vi "Drive Test.vi"(11 "Pilot-CoPilot Gamepad Controls":T1) -> ()   [LabVIEW 2014]
uses:
  Subsystems VIs/Robot Control Outputs 2015.ctl
  Global Variables/Refnum Names.vi
panel:
  # "CB = control board"
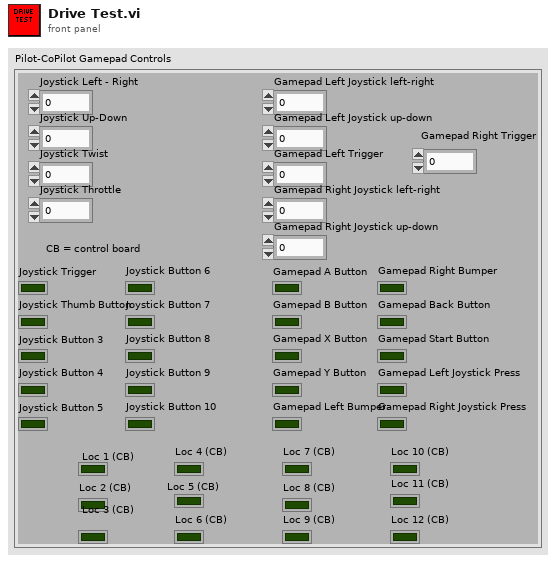
[diagram p1: front panel]
types:
  T1 = typedef "Robot Control Outputs 2015.ctl" = cluster{"Gamepad Left Joystick left-right":dbl, "Gamepad Left Joystick up-down":dbl, "Gamepad A Button":bool, "Gamepad B Button":bool, "Gamepad X Button":bool, "Gamepad Y Button":bool, "Gamepad Left Bumper":bool, "Gamepad Right Bumper":bool, "Gamepad Back Button":bool, "Gamepad Start Button":bool, "Gamepad Left Joystick Press":bool, "Gamepad Right Joystick Press":bool, "Joystick Trigger":bool, "Joystick Thumb Button":bool, "Joystick Button 3":bool, "Joystick Button 4":bool, "Joystick Button 5":bool, "Joystick Button 6":bool, "Joystick Button 7":bool, "Joystick Button 8":bool, "Joystick Button 9":bool, "Joystick Button 10":bool, "Gamepad Left Trigger":dbl, "Gamepad Right Joystick left-right":dbl, "Gamepad Right Joystick up-down":dbl, "Joystick Left - Right":dbl, "Joystick Up-Down":dbl, "Joystick Twist":dbl, "Joystick Throttle":dbl, "Loc 1 (CB)":bool, "Loc 4 (CB)":bool, "Gamepad Right Trigger":dbl, "Loc 2 (CB)":bool, "Loc 3 (CB)":bool, "Loc 5 (CB)":bool, "Loc 6 (CB)":bool, "Loc 7 (CB)":bool, "Loc 10 (CB)":bool, "Loc 8 (CB)":bool, "Loc 9 (CB)":bool, "Loc 11 (CB)":bool, "Loc 12 (CB)":bool}
  T2 = typedef "WPI_MotorControlDeviceRef.ctl" = cluster{"DeviceStatus":errorcluster, "Type":T3, "PWM":cluster{"Controller":T4, "PWM Channel":T5, "DeadBand":T6}, "CAN":cluster{"Device Number":u8, "Control Mode":T7, "Semaphore":T8, "Max Vout":dbl, "TalonSRX Control Mode":T9}, "Invert":bool, "TransformRef":T10, "InvTransformRef":T10}
  T3 = typedef "WPI_MotorControlType.ctl" = enum16{"PWM", "CAN", "CANTalonSRX"}
  T4 = typedef "FPGA_TypedefDigitalModule.ctl" = enum16{"Controller 1"}
  T5 = typedef "FPGA_DIOPWMChannel.ctl" = enum8{"PWM 0", "PWM 1", "PWM 2", "PWM 3", "PWM 4", "PWM 5", "PWM 6", "PWM 7", "PWM 8", "PWM 9", "PWM MXP 0", "PWM MXP 1", "PWM MXP 2", "PWM MXP 3", "PWM MXP 4", "PWM MXP 5", "PWM MXP 6", "PWM MXP 7", "PWM MXP 8", "PWM MXP 9", "Invalid"}
  T6 = typedef "WPI_PWMDeadband.ctl" = cluster{"Name":string, "maxPositivePwm":i32, "minPositivePwm":i32, "centerPwm":i32, "maxNegativePwm":i32, "minNegativePwm":i32, "angularRange":u16}
  T7 = typedef "WPI_CANJaguar_ControlMode.ctl" = enum8{"Percent VBus", "Current", "Speed", "Position", "Voltage"}
  T8 = typedef "Semaphore RefNum" = refnum<k1>
  T9 = typedef "WPI_CANTalonSRX_APIControlMode.ctl" = enum8{"Percent VBus", "Speed", "Position", "Slave", "Unchanged / Invalid"}
  T10 = typedef "WPI_PWMTransform_ConPane.ctl" = refnum<vi>
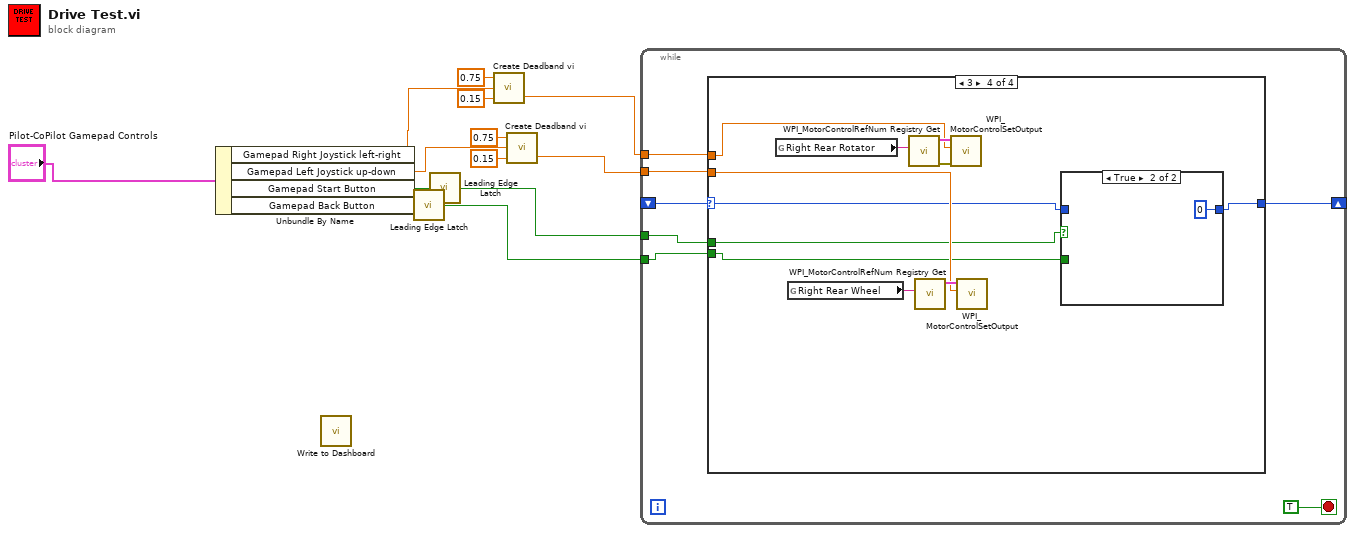
[diagram p0: block diagram]
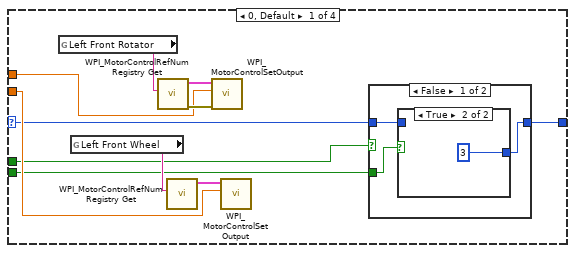
[diagram p2: hidden frame]
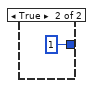
[diagram p4: hidden frame]
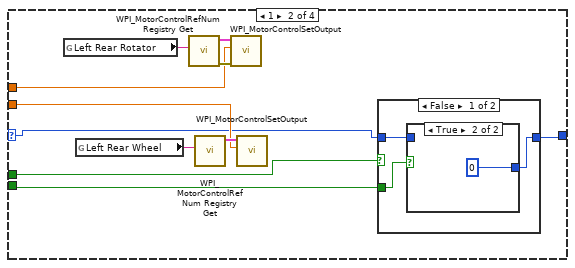
[diagram p5: hidden frame]
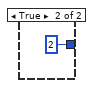
[diagram p7: hidden frame]
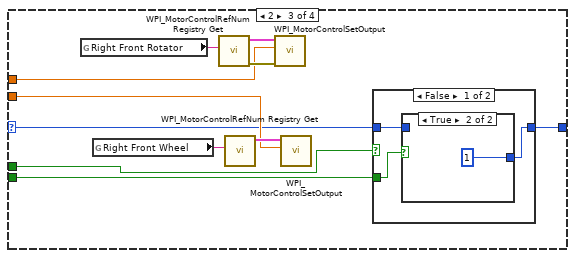
[diagram p8: hidden frame]
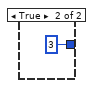
[diagram p10: hidden frame]
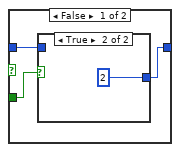
[diagram p11: hidden frame]
diagram:
  n1 = Unbundle By Name("Pilot-CoPilot Gamepad Controls") -> ("Gamepad Right Joystick left-right"=w8:dbl, "Gamepad Left Joystick up-down"=w2:dbl, "Gamepad Start Button"=w12:bool, "Gamepad Back Button"=w11:bool)
  n2 = call "Write to Dashboard.vi"() -> ()  [unwired: 12 in]
  n3 = call "Leading Edge Latch.vi"("Input"=w11) -> ("Output"=w10:bool)
  n4 = call "Leading Edge Latch.vi"("Input"=w12) -> ("Output"=w9:bool)
  n5 = call "Create Deadband vi.vi"("Input Deadband"=0.15, "Input"=w8, "Output Upper Limit"=0.75) -> ("Output"=w5:dbl)  [unwired: 1 in]
  n6 = call "Create Deadband vi.vi"("Input Deadband"=0.15, "Input"=w2, "Output Upper Limit"=0.75) -> ("Output"=w1:dbl)  [unwired: 1 in]
  n7 = while {
    tunnel: w5 -> [w20]
    tunnel: w1 -> [w19]
    shift-right: [w17] -> _
    shift-left: _ -> [w16]
    tunnel: w9 -> [w15]
    tunnel: w10 -> [w14]
    stop <- TRUE stop-if-true
    n8 = case shown="3" w16 {
      selector: w16 -> [w23 w38 w57 w74]
      tunnel: w20 -> [w26 w43 w60 w77]
      tunnel: w19 -> [w25 w42 w59 w76]
      tunnel: [w22 w41 w58 w75] -> w17
      tunnel: w15 -> [w24 w39 w56 w73]
      tunnel: w14 -> [w21 w40 w55 w72]
      frame 0, Default {
        n9 = global read "Refnum Names.vi" "Left Front Rotator"() -> (w31:string)
        n10 = global read "Refnum Names.vi" "Left Front Wheel"() -> (w28:string)
        n11 = call <vilib>:"WPI_MotorControlRefNum Registry Get.vi"("refnum name"=w31) -> ("error out"=w29:errorcluster, "MotorControlDevRef"=w30:T2)  [unwired: 9 in]
        n12 = call <vilib>:"WPI_MotorControlRefNum Registry Get.vi"("refnum name"=w28) -> ("MotorControlDevRef"=w27:T2)  [unwired: 9 in, 1 out]
        n13 = call <vilib>:"WPI_MotorControlSetOutput.vi"("error in (no error)"=w29, "Output"=w26, "MotorControlDevRef"=w30) -> ()  [unwired: 6 in, 3 out]
        n14 = call <vilib>:"WPI_MotorControlSetOutput.vi"("Output"=w25, "MotorControlDevRef"=w27) -> ()  [unwired: 7 in, 3 out]
        n15 = case shown="False" w24 {
          tunnel: w23 -> [w32 _]
          tunnel: [w33 1] -> w22
          tunnel: w21 -> [w34 _]
          frame False {
            n16 = case shown="True" w34 {
              tunnel: [w35 3] -> w33
              tunnel: w32 -> [w35 _]
              frame False {
              }
              frame True {
              }
            }
          }
          frame True {
          }
        }
      }
      frame 1 {
        n17 = global read "Refnum Names.vi" "Left Rear Rotator"() -> (w48:string)
        n18 = global read "Refnum Names.vi" "Left Rear Wheel"() -> (w45:string)
        n19 = call <vilib>:"WPI_MotorControlRefNum Registry Get.vi"("refnum name"=w48) -> ("error out"=w46:errorcluster, "MotorControlDevRef"=w47:T2)  [unwired: 9 in]
        n20 = call <vilib>:"WPI_MotorControlRefNum Registry Get.vi"("refnum name"=w45) -> ("MotorControlDevRef"=w44:T2)  [unwired: 9 in, 1 out]
        n21 = call <vilib>:"WPI_MotorControlSetOutput.vi"("error in (no error)"=w46, "Output"=w43, "MotorControlDevRef"=w47) -> ()  [unwired: 6 in, 3 out]
        n22 = call <vilib>:"WPI_MotorControlSetOutput.vi"("Output"=w42, "MotorControlDevRef"=w44) -> ()  [unwired: 7 in, 3 out]
        n23 = case shown="False" w39 {
          tunnel: w38 -> [w49 _]
          tunnel: [w50 2] -> w41
          tunnel: w40 -> [w51 _]
          frame False {
            n24 = case shown="True" w51 {
              tunnel: [w52 0] -> w50
              tunnel: w49 -> [w52 _]
              frame False {
              }
              frame True {
              }
            }
          }
          frame True {
          }
        }
      }
      frame 2 {
        n25 = global read "Refnum Names.vi" "Right Front Rotator"() -> (w65:string)
        n26 = global read "Refnum Names.vi" "Right Front Wheel"() -> (w62:string)
        n27 = call <vilib>:"WPI_MotorControlRefNum Registry Get.vi"("refnum name"=w65) -> ("error out"=w63:errorcluster, "MotorControlDevRef"=w64:T2)  [unwired: 9 in]
        n28 = call <vilib>:"WPI_MotorControlRefNum Registry Get.vi"("refnum name"=w62) -> ("MotorControlDevRef"=w61:T2)  [unwired: 9 in, 1 out]
        n29 = call <vilib>:"WPI_MotorControlSetOutput.vi"("error in (no error)"=w63, "Output"=w60, "MotorControlDevRef"=w64) -> ()  [unwired: 6 in, 3 out]
        n30 = call <vilib>:"WPI_MotorControlSetOutput.vi"("Output"=w59, "MotorControlDevRef"=w61) -> ()  [unwired: 7 in, 3 out]
        n31 = case shown="False" w56 {
          tunnel: w57 -> [w66 _]
          tunnel: [w67 3] -> w58
          tunnel: w55 -> [w68 _]
          frame False {
            n32 = case shown="True" w68 {
              tunnel: [w69 1] -> w67
              tunnel: w66 -> [w69 _]
              frame False {
              }
              frame True {
              }
            }
          }
          frame True {
          }
        }
      }
      frame 3 {
        n33 = global read "Refnum Names.vi" "Right Rear Rotator"() -> (w82:string)
        n34 = global read "Refnum Names.vi" "Right Rear Wheel"() -> (w79:string)
        n35 = call <vilib>:"WPI_MotorControlRefNum Registry Get.vi"("refnum name"=w82) -> ("error out"=w80:errorcluster, "MotorControlDevRef"=w81:T2)  [unwired: 9 in]
        n36 = call <vilib>:"WPI_MotorControlRefNum Registry Get.vi"("refnum name"=w79) -> ("MotorControlDevRef"=w78:T2)  [unwired: 9 in, 1 out]
        n37 = call <vilib>:"WPI_MotorControlSetOutput.vi"("error in (no error)"=w80, "Output"=w77, "MotorControlDevRef"=w81) -> ()  [unwired: 6 in, 3 out]
        n38 = call <vilib>:"WPI_MotorControlSetOutput.vi"("Output"=w76, "MotorControlDevRef"=w78) -> ()  [unwired: 7 in, 3 out]
        n39 = case shown="True" w73 {
          tunnel: w74 -> [w83 _]
          tunnel: [w84 0] -> w75
          tunnel: w72 -> [w85 _]
          frame False {
            n40 = case shown="True" w85 {
              tunnel: [w86 2] -> w84
              tunnel: w83 -> [w86 _]
              frame False {
              }
              frame True {
              }
            }
          }
          frame True {
          }
        }
      }
    }
  }
